vi "Robot Global Data.vi"() -> ()   [LabVIEW 2012]
doc: "This global VI can contain as many global variables as you need. Place a control on the panel, give it a good name. To read or write to it from a VI, drag the icon to the diagram of that VI. You can also drag from the project. Click on the node to change which global you access. You shouldn't have multiple locations writing to a global or it will cause a race-condition."
uses:
  <vilib>/Rock Robotics/WPI/Camera/WPI_CameraImageSize.ctl
  <vilib>/Rock Robotics/WPI/DriverStation/WPI_DriverStationRobotMode2.ctl
panel:
  out "Current File":dbl
  out "Circle Info":cluster{dbl, dbl}
  out "ShootOutFlipper":dbl
  out "ShootOutRollers":dbl
  out "ShootOutWheelF":dbl
  out "ShootOutElev":dbl
  out "ShootOutIndexer":dbl
  in  "ShootTrackEnable":bool
  in  "ShootStartWheels":bool
  in  "ShootIndexerEnable":bool
  in  "ShootCase":dbl
  in  "ShootManualElev":dbl
  in  "ShootIndexerSpd":dbl=0.5
  in  "ShootWheelSpd":dbl=0.7
  in  "ShootConstElev":T1={"Ground"=4.0, "1"=3.5, "2"=3.0, "3"=2.5, "4"=2.0}
  in  "ShootRollerSpd":dbl
  in  "ShootConstFlipper":cluster{"Down":dbl, "Up":dbl}={"Down"=0.2, "Up"=0.8}
  out "Target Info":cluster{"X":dbl, "Y":dbl, "Distance (ft)":dbl}
  in  "Servo Positions":T2={"Shifting"={"Right Servo High"=145.0, "Right Servo Low"=110.0, "Left Servo High"=70.0, "Left Servo Low"=110.0}, "Breaking"={"Coast Position"=0.0, "Break Position"=0.0}}
  out "Auton Array":dbl[][](array[numeric]) format="%0.3f"
  out "Auton Files":string[](array[string])
  out "Number of Auton Files":dbl
  in  "Robot Mode":T3
  in  "LED toggle rate (ms)":u32=20
  in  "image size":T4=enum."320x240"
  in  "Enable Vision":bool
  # "Shoot Globals"
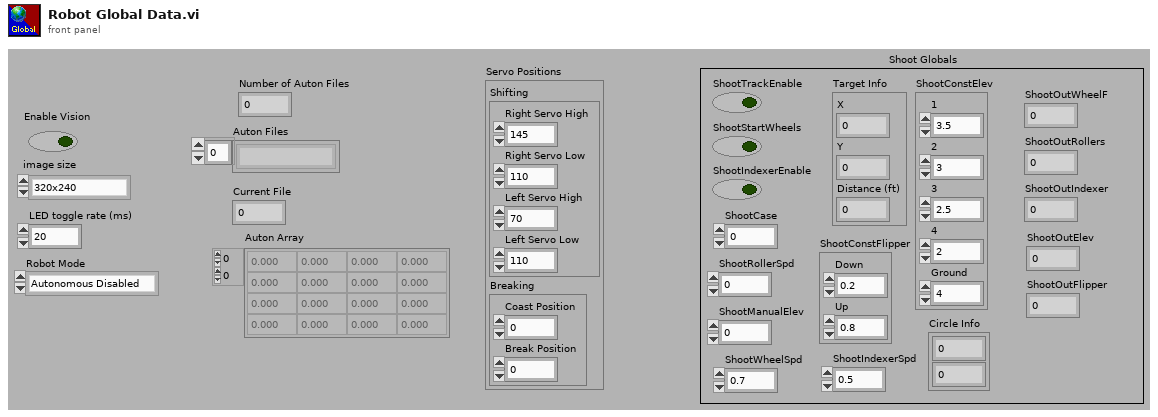
[diagram p1: front panel]
types:
  T1 = cluster{"Ground":dbl, "1":dbl, "2":dbl, "3":dbl, "4":dbl}
  T2 = cluster{"Shifting":cluster{"Right Servo High":dbl, "Right Servo Low":dbl, "Left Servo High":dbl, "Left Servo Low":dbl}, "Breaking":cluster{"Coast Position":dbl, "Break Position":dbl}}
  T3 = typedef "WPI_DriverStationRobotMode2.ctl" = enum16{"Autonomous Disabled", "Autonomous Enabled", "Teleop Disabled", "Teleop Enabled", "Timeout", "Finish", "Test Disabled", "Test Enabled"}
  T4 = typedef "WPI_CameraImageSize.ctl" = enum16{"640x480", "320x240", "160x120"}
diagram:
